vi "user input.vi"(8 "error in":errorcluster) -> (0 "error out":errorcluster, 3 "Inputs from system":T1)   [LabVIEW 2017, in "ActiveFrontEndModule runtime.lvclass"]
uses:
  ActiveFrontEndModule runtime.lvclass
  input user data.ctl
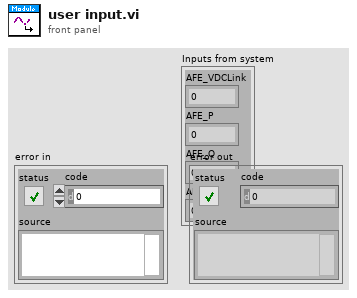
[diagram p1: front panel]
types:
  T1 = typedef "ActiveFrontEndModule runtime.lvclass/input user data.ctl" = cluster{"AFE_VDCLink":dbl, "AFE_P":dbl, "AFE_Q":dbl, "AFE_pf":dbl}
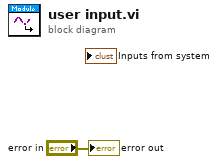
[diagram p0: block diagram]
diagram:
  "error out" <- "error in"
